vi "test Parse Sorted Object Dictionary_1.vi"(11 "Test Case In":refnum<class "test Electronic Datasheet.lvclass">) -> (0 "error out":errorcluster, 3 "Test Case Out":refnum<class "test Electronic Datasheet.lvclass">)   [LabVIEW 2024, in "test Electronic Datasheet.lvclass"]
uses:
  test Electronic Datasheet.lvclass
  C:/Program Files/National Instruments/LabVIEW 2024/vi.lib/Astemes/LUnit/Test Case.lvclass
  Core/Object Type.ctl
  Core/Data Type.ctl
  Core/Access Type.ctl
  <vilib>/Astemes/LUnit/Test Case.lvclass/Test Case.ctl
  <vilib>/Astemes/LUnit/Append Fail Result.vi
  <vilib>/Astemes/LUnit/Append Pass Result.vi
  <vilib>/Astemes/LUnit/Run In UI.vi
  <vilib>/Utility/error.llb/Clear Errors.vi
  Core/OD Sub-Entry/OD Sub-Entry.lvclass
  D:/git/EDS-File-Viewer/Core/OD Entry/OD Entry.lvclass
  Electronic Datasheet/utils/Electronic Datasheet_GetAttributes.vi
  Electronic Datasheet/Electronic Datasheet.lvclass
  <vilib>/Astemes/LUnit/Test Case.lvclass
  Core/Electronic Datasheet.lvlib
  Core/OD Entry/OD Entry.lvclass
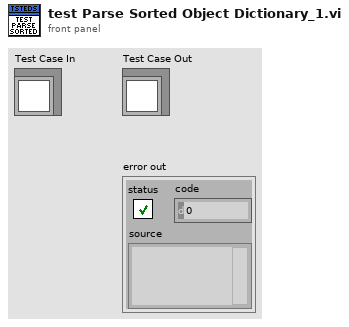
[diagram p1: front panel]
types:
  T1 = typedef "Electronic Datasheet.lvlib/Access Type.ctl" = enum16{"ro", "wo", "rw", "rwr", "rww", "const"}
  T2 = typedef "Electronic Datasheet.lvlib/Data Type.ctl" = u16
  T3 = typedef "Electronic Datasheet.lvlib/Object Type.ctl" = u8
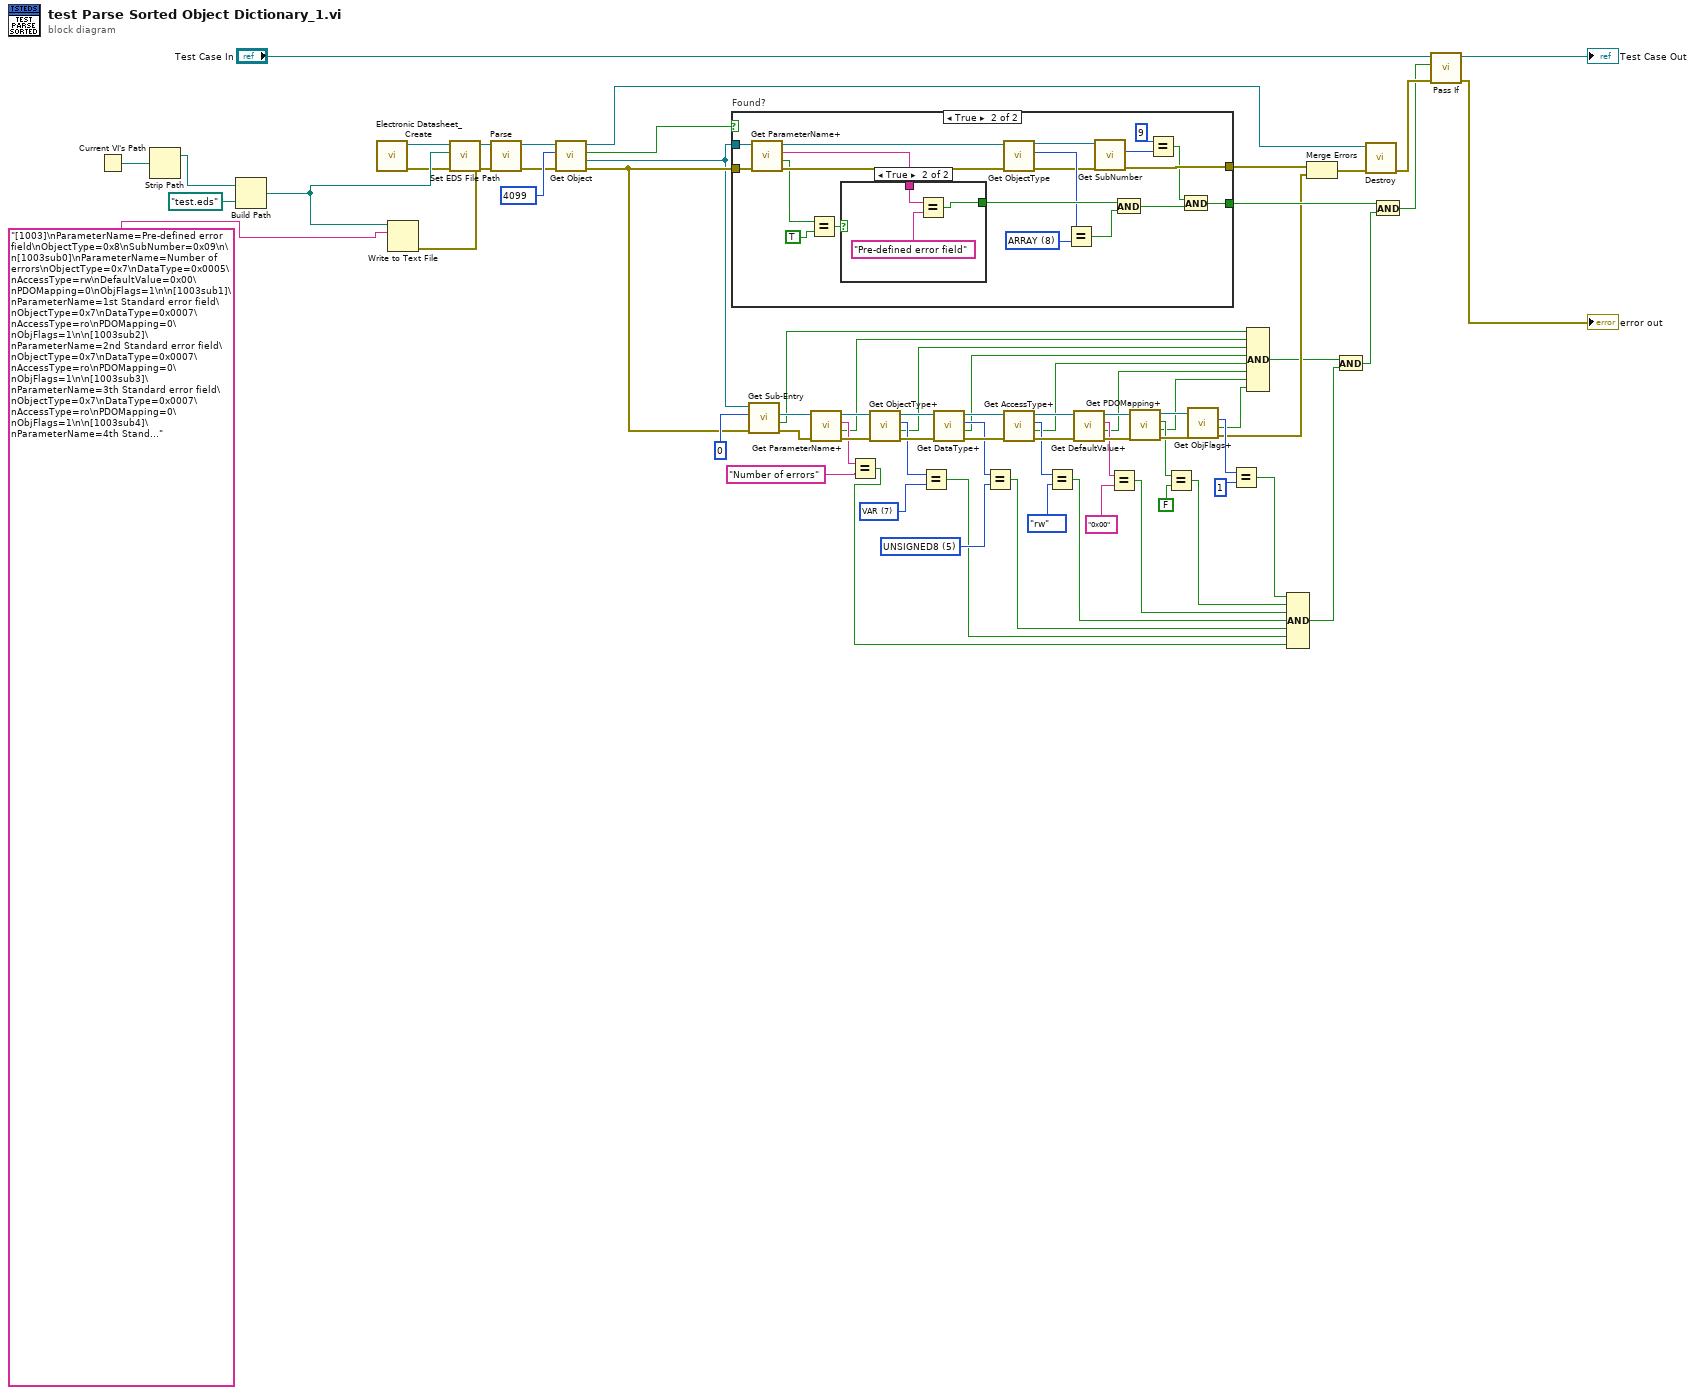
[diagram p0: block diagram]
diagram:
  w41 = T2 5 items=["BOOLEAN"=1, "INTEGER8"=2, "INTEGER16"=3, "INTEGER32"=4, "UNSIGNED8"=5, "UNSIGNED16"=6, "UNSIGNED32"=7, "REAL32"=8, "VISIBLE_STRING"=9, "OCTET_STRING"=10, "UNICODE_STRING"=11, "TIME_OF_DAY"=12, "TIME_DIFFERENCE"=13, "RESERVED1"=14, "DOMAIN"=15, "INTEGER24"=16, "REAL64"=17, "INTEGER40"=18, "INTEGER48"=19, "INTEGER56"=20, "INTEGER64"=21, "UNSIGNED24"=22, "RESERVED2"=23, "UNSIGNED40"=24, "UNSIGNED48"=25, "UNSIGNED56"=26, "UNSIGNED64"=27, "RESERVED3"=28, "RESERVED4"=29, "RESERVED5"=30, "RESERVED6"=31, "PDO_COMMUNICATION_PARAMETER"=32, "PDO_MAPPING"=33, "SDO_PARAMETER"=34, "IDENTITY"=35, "RESERVED7"=36] ("DataType")
  w43 = T3 7 items=["NULL"=0, "DOMAIN"=2, "DEFTYPE"=5, "DEFSTRUCT"=6, "VAR"=7, "ARRAY"=8, "RECORD"=9] ("ObjectType")
  n1 = Current VI's Path() -> (path=w68:path)
  n2 = Strip Path(path=w68) -> (stripped path=w64:path)  [unwired: 1 out]
  n3 = Build Path(base path=w64, name or relative path=path "test.eds") -> (appended path=w65:path)
  n4 = call "Electronic Datasheet_Create.vi"() -> ("Error Out"=w7:errorcluster, "reference out"=w8:refnum<class "Electronic Datasheet.lvclass">)  [unwired: 10 in]
  n5 = Write to Text File(file (use dialog)=w65, text="[1003]\nParameterName=Pre-defined error field\nObjectType=0x8\nSubNumber=0x09\n\n[1003sub0]\nParameterName=Number of errors\nObjectType=0x7\nDataType=0x0005\nAccessType=rw\nDefaultValue=0x00\nPDOMapping=0\nObjFlags=1\n\n[1003sub1]\nParameterName=1st Standard error field\nObjectType=0x7\nDataType=0x0007\nAccessType=ro\nPDOMapping=0\nObjFlags=1\n\n[1003sub2]\nParameterName=2nd Standard error field\nObjectType=0x7\nDataType=0x0007\nAccessType=ro\nPDOMapping=0\nObjFlags=1\n\n[1003sub3]\nParameterName=3th Standard error field\nObjectType=0x7\nDataType=0x0007\nAccessType=ro\nPDOMapping=0\nObjFlags=1\n\n[1003sub4]\nParameterName=4th Standard error field\nObjectType=0x7\nDataType=0x0007\nAccessType=ro\nPDOMapping=0\nObjFlags=1\n\n[1003sub5]\nParameterName=5th Standard error field\nObjectType=0x7\nDataType=0x0007\nAccessType=ro\nPDOMapping=0\nObjFlags=1\n\n[1003sub6]\nParameterName=6th Standard error field\nObjectType=0x7\nDataType=0x0007\nAccessType=ro\nPDOMapping=0\nObjFlags=1\n\n[1003sub7]\nParameterName=7th Standard error field\nObjectType=0x7\nDataType=0x0007\nAccessType=ro\nPDOMapping=0\nObjFlags=1\n\n[1003sub8]\nParameterName=8th Standard error field\nObjectType=0x7\nDataType=0x0007\nAccessType=ro\nPDOMapping=0\nObjFlags=1") -> (error out=w66:errorcluster)  [unwired: 2 in, 2 out]
  n6 = call "Set EDS File Path.vi"("error in"=w7, "EDS File Path"=w65, "reference in"=w8) -> ("reference out"=w69:refnum<class "Electronic Datasheet.lvclass">)  [unwired: 7 in, 1 out]
  n7 = call "Parse.vi"("error in"=w66, "reference in"=w69) -> ("error out"=w5:errorcluster, "reference out"=w63:refnum<class "Electronic Datasheet.lvclass">)  [unwired: 8 in]
  n8 = call "Get Object.vi"("error in"=w5, "Index"=u16 4099 ("Numeric"), "reference in"=w63) -> ("error out"=w4:errorcluster, "OD Entry"=w1:refnum<class "OD Entry.lvclass">, "Found?"=w2:bool, "reference out"=w3:refnum<class "Electronic Datasheet.lvclass">)  [unwired: 5 in]
  n9 = case "Found?" shown="True" w2 {
    selector: w2 -> [w73 _]
    tunnel: w1 -> [_ w94]
    tunnel: w4 -> [w74 w93]
    tunnel: [w73 w77] -> w61
    tunnel: [w74 w81] -> w59
    frame False {
    }
    frame True {
      w85 = T3 8 items=["NULL"=0, "DOMAIN"=2, "DEFTYPE"=5, "DEFSTRUCT"=6, "VAR"=7, "ARRAY"=8, "RECORD"=9] ("y")
      n10 = call "Get ParameterName+.vi"("Error In"=w93, "reference in"=w94) -> ("Error Out"=w87:errorcluster, "Defined?"=w75:bool, "ParameterName"=w91:string, "reference out"=w88:refnum<class "OD Entry.lvclass">)  [unwired: 6 in]
      n11 = Equal?(x=w75, y=TRUE) -> (x = y?=w90:bool)
      n12 = case shown="True" w90 {
        selector: w90 -> [w95 _]
        tunnel: w91 -> [_ w98]
        tunnel: [w95 w96] -> w89
        frame False {
        }
        frame True {
          n13 = Equal?(x=w98, y="Pre-defined error field") -> (x = y?=w96:bool)
        }
      }
      n14 = call "Get ObjectType.vi"("Error In"=w87, "reference in"=w88) -> ("Error Out"=w82:errorcluster, "ObjectType"=w86:T3, "reference out"=w80:refnum<class "OD Entry.lvclass">)  [unwired: 7 in]
      n15 = Equal?(x=w86, y=w85) -> (x = y?=w83:bool)
      n16 = call "Get SubNumber.vi"("Error In"=w82, "reference in"=w80) -> ("Error Out"=w81:errorcluster, "SubNumber"=w79:u8)  [unwired: 6 in, 2 out]
      n17 = And(x=w89, y=w83) -> (x .and. y?=w84:bool)
      n18 = Equal?(x=u8 9, y=w79) -> (x = y?=w76:bool)
      n19 = And(x=w76, y=w84) -> (x .and. y?=w77:bool)
    }
  }
  n20 = call "Get Sub-Entry.vi"("Error In"=w4, "Sub-Index"=u8 0, "reference in"=w1) -> ("Error Out"=w57:errorcluster, "Found?"=w45:bool, "OD Sub-Entry"=w58:refnum<class "OD Sub-Entry.lvclass">)  [unwired: 5 in, 1 out]
  n21 = call "Get ParameterName+.vi"("Error In"=w57, "reference in"=w58) -> ("Error Out"=w56:errorcluster, "Defined?"=w15:bool, "ParameterName"=w47:string, "reference out"=w55:refnum<class "OD Sub-Entry.lvclass">)  [unwired: 6 in]
  n22 = Equal?(x=w47, y="Number of errors") -> (x = y?=w22:bool)
  n23 = call "Get ObjectType+.vi"("Error In"=w56, "reference in"=w55) -> ("Error Out"=w53:errorcluster, "Defined?"=w14:bool, "ObjectType"=w44:T3, "reference out"=w54:refnum<class "OD Sub-Entry.lvclass">)  [unwired: 6 in]
  n24 = Equal?(x=w44, y=w43) -> (x = y?=w21:bool)
  n25 = call "Get DataType+.vi"("Error In"=w53, "reference in"=w54) -> ("Error Out"=w50:errorcluster, "Defined?"=w13:bool, "DataType"=w42:T2, "reference out"=w51:refnum<class "OD Sub-Entry.lvclass">)  [unwired: 6 in]
  n26 = Equal?(x=w42, y=w41) -> (x = y?=w20:bool)
  n27 = call "Get AccessType+.vi"("Error In"=w50, "reference in"=w51) -> ("Error Out"=w48:errorcluster, "Defined?"=w12:bool, "AccessType"=w40:T1, "reference out"=w49:refnum<class "OD Sub-Entry.lvclass">)  [unwired: 6 in]
  n28 = Equal?(x=w40, y=Access_Type."rw") -> (x = y?=w19:bool)
  n29 = call "Get DefaultValue+.vi"("Error In"=w48, "reference in"=w49) -> ("Error Out"=w37:errorcluster, "Defined?"=w11:bool, "DefaultValue"=w34:string, "reference out"=w38:refnum<class "OD Sub-Entry.lvclass">)  [unwired: 6 in]
  n30 = Equal?(x=w34, y="0x00") -> (x = y?=w18:bool)
  n31 = call "Get PDOMapping+.vi"("Error In"=w37, "reference in"=w38) -> ("Error Out"=w35:errorcluster, "Defined?"=w10:bool, "PDOMapping"=w32:bool, "reference out"=w36:refnum<class "OD Sub-Entry.lvclass">)  [unwired: 6 in]
  n32 = Equal?(x=w32, y=FALSE) -> (x = y?=w17:bool)
  n33 = call "Get ObjFlags+.vi"("Error In"=w35, "reference in"=w36) -> ("Error Out"=w28:errorcluster, "Defined?"=w9:bool, "ObjFlags"=w30:u32)  [unwired: 6 in, 1 out]
  n34 = Equal?(x=w30, y=u32 1) -> (x = y?=w16:bool)
  n35 = Compound Arithmetic op=AND(w45, w15, w14, w13, w12, w11, w10, w9) -> (w26:bool)
  n36 = Compound Arithmetic op=AND(w16, w17, w18, w19, w20, w21, w22) -> (w23:bool)
  n37 = Merge Errors(w59, w28) -> (w29:errorcluster)
  n38 = And(x=w26, y=w23) -> (x .and. y?=w24:bool)
  n39 = call-dynamic "Destroy.vi"("Error In"=w29, "reference in"=w3) -> ("Error Out"=w60:errorcluster)  [unwired: 8 in, 1 out]
  n40 = And(x=w61, y=w24) -> (x .and. y?=w27:bool)
  n41 = call <vilib>:"Pass If.vi"("error in (no error)"=w60, "Pass?"=w27, "LUnit Test Case In"="Test Case In") -> ("error out"=→"error out":errorcluster, "LUnit Test Case Out"=→"Test Case Out":refnum<class "test Electronic Datasheet.lvclass">)  [unwired: 7 in]
